vi "wait for new data from server.vi"() -> (3 "Letture":T1 {"Stato uscite"."AO" format="%f%0.2f"; "AI2" format="%#_6f"; "TC" format="%#_4f"; "AI1" format="%#_6f"})   [LabVIEW 2019]
uses:
  Pedrollo Server/TypeDef/IN_Cluster.ctl
  Pedrollo Server/TypeDef/OUT_CLUSTER.ctl
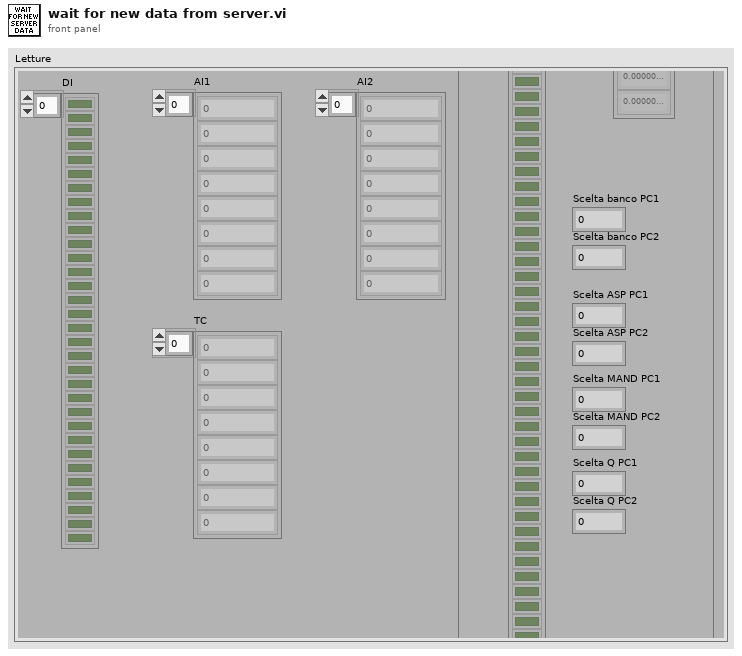
[diagram p1: front panel]
types:
  T1 = typedef "IN_Cluster.ctl" = cluster{"DI":bool[], "AI1":dbl[], "TC":dbl[], "AI2":dbl[], "Stato uscite":T2}
  T2 = typedef "OUT_CLUSTER.ctl" = cluster{"DO ":bool[], "AO":dbl[], "Scelta banco PC1":dbl, "Scelta banco PC2":dbl, "Scelta ASP PC1":dbl, "Scelta ASP PC2":dbl, "Scelta MAND PC1":dbl, "Scelta MAND PC2":dbl, "Scelta Q PC1":dbl, "Scelta Q PC2":dbl}
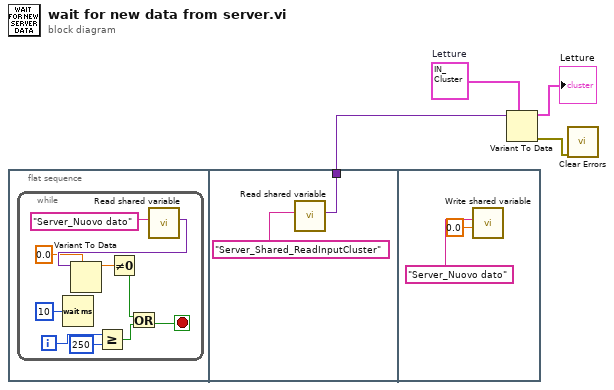
[diagram p0: block diagram]
diagram:
  w2 = T1 {"DI"=[], "AI1"=[], "TC"=[], "AI2"=[], "Stato uscite"={"DO "=[], "AO"=[], "Scelta banco PC1"=0.0, "Scelta banco PC2"=0.0, "Scelta ASP PC1"=0.0, "Scelta ASP PC2"=0.0, "Scelta MAND PC1"=0.0, "Scelta MAND PC2"=0.0, "Scelta Q PC1"=0.0, "Scelta Q PC2"=0.0}}  # Letture
  n1 = flat-sequence {
    tunnel: [w16] -> w4
    frame #0 {
      n2 = while {
        i -> [w13]
        stop <- w11 stop-if-true
        n3 = Wait (ms)(milliseconds to wait=u32 10) -> ()  [unwired: 1 out]
        n4 = Greater Or Equal?(x=w13, y=250) -> (x >= y?=w10:bool)
        n5 = call "Read shared variable.vi"("nome shared variable"="Server_Nuovo dato") -> ("lettura"=w8:variant)  [unwired: 9 in, 1 out]
        n6 = Variant To Data(type=0.0, Variant=w8) -> (data=w6:dbl)  [unwired: 1 in, 1 out]
        n7 = Not Equal To 0?(x=w6) -> (x != 0?=w5:bool)
        n8 = Or(x=w5, y=w10) -> (x .or. y?=w11:bool)
      }
    }
    frame #1 {
      n9 = call "Read shared variable.vi"("nome shared variable"="Server_Shared_ReadInputCluster") -> ("lettura"=w16:variant)  [unwired: 9 in, 1 out]
    }
    frame #2 {
      n10 = call "Write shared variable.vi"("DATO DBL"=0.0, "nome shared variable"="Server_Nuovo dato") -> ()  [unwired: 9 in, 1 out]
    }
  }
  n11 = Variant To Data(type=w2, Variant=w4) -> (data=→"Letture":T1, error out=w1:errorcluster)  [unwired: 1 in]
  n12 = call <vilib>:"Clear Errors.vi"("error in (no error)"=w1) -> ()  [unwired: 5 in, 2 out]
